vi "AuMT8852B User Text.vi"(5 "User text (\"\")":string, 7 "Set/Get (Set)":enum16{"Set", "Get"}(ring), 8 "error in (no error)":errorcluster, 11 "VISA session":refnum<visa-resource-name>) -> (0 "error out":errorcluster, 2 "error code":i32, 3 "VISA session out":refnum<visa-resource-name>, 4 "User text out":string)   [LabVIEW 2017]
doc: "Anritsu MT8852B Bluetooth Tester\n\nSets or queries a user-definable string to be displayed on the instrument.\n\nINPUTS\nSet/Get - whether the value is being sent to or retrieved from the instrument.\nUser text - information (20 characters max) to send to the instrument.\n\nOUTPUTS\nUser text out - information to be retrieved from the instrument"
uses:
  <instrlib>/aumt8852B/General/Utilities/MT8850 Attribute ID.ctl
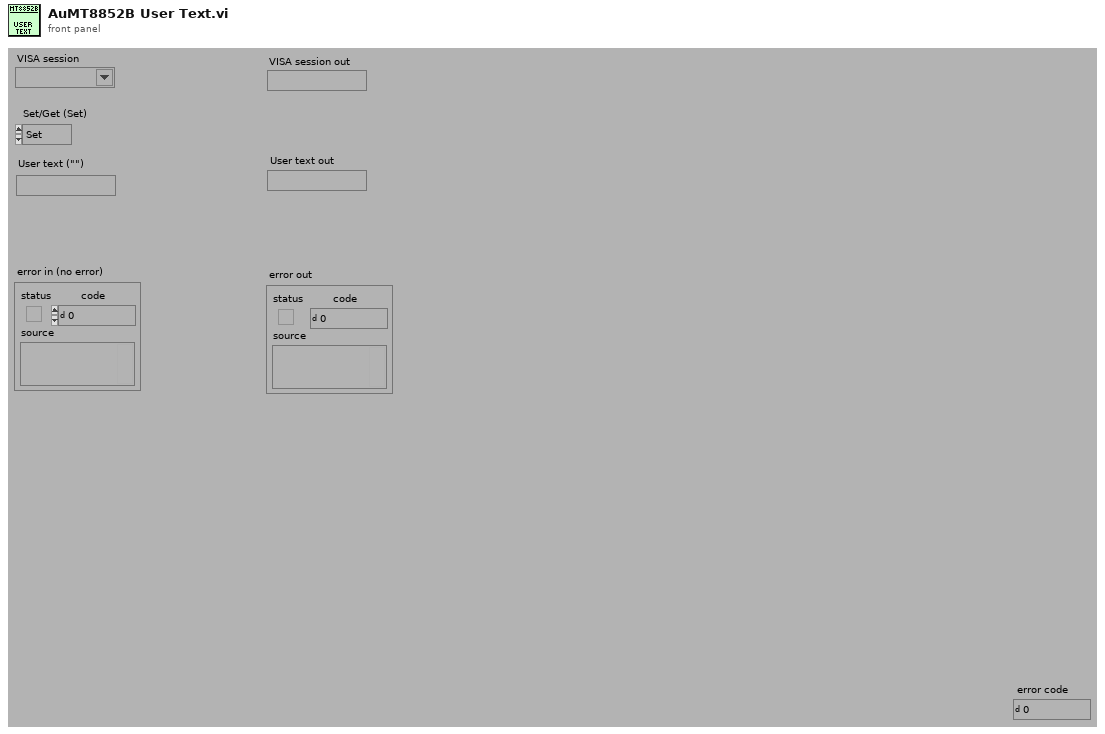
[diagram p1: front panel]
types:
  T1 = typedef "MT8850 Attribute ID.ctl" = enum16{"Operation mode", "Selected script", "EUT address source", "EUT Address", "EUT HCI RS232 Baud Rate", "Tester GPIB Address", "Tester RS232 Baud Rate", "Tester Bluetooth Address", "Tester Contrast", "Tester Key Click On", "Tester Modulation Index", "Tester Poll-Null Mode", "Tester Power Range", "Tester RS232 Mode", "Beep on Illegal Entry", "Display User Text", "User Text", "Calibration TX Modulation DAC", "Calibration RX Channel", "Calibration TX Channel", "Calibration TX Power", "Calibration Use TX Table", "Inquiry Request User-friendly Name", "Inquiry Number of Responses", "Inquiry Timeout", "Script Frequency Display", "Script Loop Count", "Script Loop Continuously", "Script Loop Stop on Fail", "Link timeout", "Page timeout", "Filter bandwidth", "SCO air code", "SCO bit position", "SCO input code", "SCO input data", "SCO input sample size", "SCO loopback mode", "SCO packet type", "SCO tone generator", "Tester page scan repetition mode", "Tester follow test mode", "Tester authentication state", "Tester authentication pin code", "Tester authentication pin length"}
  T2 = typedef "Attribute Status.ctl" = enum16{"No I/O needed", "I/O needed"}
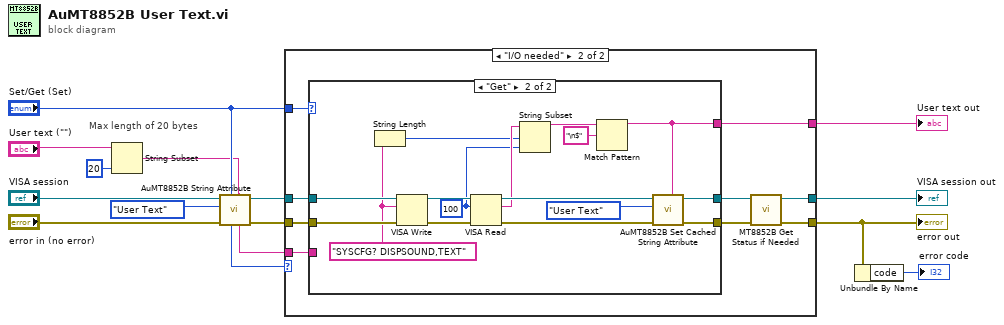
[diagram p0: block diagram]
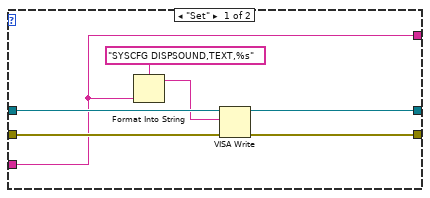
[diagram p3: hidden frame]
diagram:
  # "Max length of 20 bytes"
  n1 = String Subset(string="User text (\"\")", length (rest)=20 ("length (rest)")) -> (substring=w3:string)  [unwired: 1 in]
  n2 = call <instrlib>:"AuMT8852B String Attribute.vi"("Value (\"\")"=w3, "Set/Get (Set)"="Set/Get (Set)", "error in (no error)"="error in (no error)", "Attribute ID"=MT8850_Attribute_ID."User Text", "VISA session"="VISA session") -> ("error out"=w11:errorcluster, "VISA session out"=w12:refnum<visa-resource-name>, "Value out"=w14:string, "Status"=w10:T2)  [unwired: 3 in]
  n3 = case shown="\"I/O needed\"" w10 {
    tunnel: "Set/Get (Set)" -> [_ w27]
    tunnel: w14 -> [w18 w26]
    tunnel: [w16 w19] -> w1
    tunnel: [w17 w20] -> w13
    tunnel: w12 -> [w17 w25]
    tunnel: w11 -> [w16 w24]
    tunnel: [w18 w23] -> w9
    frame "No I/O needed", Default {
    }
    frame "I/O needed" {
      n4 = case shown="\"Get\"" w27 {
        tunnel: [w31 w43] -> w21
        tunnel: w26 -> [w28 _]
        tunnel: [w32 w44] -> w22
        tunnel: w25 -> [w34 w50]
        tunnel: w24 -> [w33 w49]
        tunnel: [w28 w36] -> w23
        frame "Set" {
          n5 = Format Into String(format string="SYSCFG DISPSOUND,TEXT,%s" ("Format String"), w28) -> (resulting string=w29:string)  [unwired: 2 in, 1 out]
          n6 = VISA Write(VISA resource name=w34, write buffer=w29, error in (no error)=w33) -> (VISA resource name out=w32:refnum<visa-resource-name>, error out=w31:errorcluster)  [unwired: 1 out]
        }
        frame "Get" {
          w35 = u32 100 ("byte count (0)")
          w40 = "SYSCFG? DISPSOUND,TEXT" ("write buffer (\"\")")
          n7 = String Length(string=w40) -> (length=w39:i32)
          n8 = VISA Write(VISA resource name=w50, write buffer=w40, error in (no error)=w49) -> (VISA resource name out=w48:refnum<visa-resource-name>, error out=w47:errorcluster)  [unwired: 1 out]
          n9 = VISA Read(VISA resource name=w48, byte count=w35, error in (no error)=w47) -> (VISA resource name out=w46:refnum<visa-resource-name>, read buffer=w41:string, error out=w45:errorcluster)  [unwired: 1 out]
          n10 = String Subset(string=w41, offset (0)=w39, length (rest)=w35) -> (substring=w38:string)
          n11 = Match Pattern(string=w38, regular expression="\n$") -> (before substring=w36:string)  [unwired: 1 in, 3 out]
          n12 = call <instrlib>:"AuMT8852B Set Cached String Attribute.vi"("Value (\"\")"=w36, "error in (no error)"=w45, "Attribute ID"=MT8850_Attribute_ID."User Text", "VISA session"=w46) -> ("error out"=w43:errorcluster, "VISA session out"=w44:refnum<visa-resource-name>)  [unwired: 6 in]
        }
      }
      n13 = call <instrlib>:"MT8852B Get Status if Needed.vi"("error in (no error)"=w21, "VISA session"=w22) -> ("error out"=w19:errorcluster, "VISA session out"=w20:refnum<visa-resource-name>)  [unwired: 8 in]
    }
  }
  "error out" <- w1
  "VISA session out" <- w13
  "User text out" <- w9
  n14 = Unbundle By Name(w1) -> ("code"=→"error code":i32)
